vi "PRIME Detector Wait for Command to Complete.vi"(5 "Observation":T2={"Priority"=0, "ID"="", "Observer"="", "Obj Name"="", "Obj Type"="", "RA and DEC String"={"RA"="HH:MM:SS.nnn", "DEC"="DEG:arcmin:arcsec.nn"}, "Filters"=[], "Integration Time"=0.0, "Observation Status"=enum."Error", "Offsets"={"RA"=0.0, "DEC"=0.0, "ROT"=0.0}, "Images"=0, "Dither Options"={"Dither"=enum."None", "Dither Radius"=0.0, "Dither Points"=0, "Dither Phase"=0.0, "B Offset"={"RA"=0.0, "DEC"=0.0}}, "Comment 1"="", "Comment 2"=""}, 7 "Detector Config":T8={"Detector"=0, "Offsets"=[[0, 0, 0, 0, 0, 0, 0, 0, 0, 0, 0, 0, 0, 0, 0, 0, 0, 0, 0, 0, 0, 0, 0, 0, 0, 0, 0, 0, 0, 0, 0, 0]], "Detector Computer"={"Machine"="192.168.121.11", "Password"="rSL!nux23456", "FITS File Path"="", "Port"=44444, "Header Path"="", "Name"=""}, "FITS hdr template0"=path "", "FITS hdr template1"=path "", "FITS Data File Path"=path "", "FITS Detector Settings"={"Exp Time Short"=0.0, "# of Frames"=0.0, "Exp Time Long"=0.0, "# of Groups"=0.0, "Object Name"="", "Object"="", "Obs Type"="", "Image Type"="", "Observer"="", "Observer Affiliation"=""}, "Sim Folder"=path "", "Integration Mode"=enum."Ramp", "Integration Time"=0.0, "Frame Int Time"=0.0} {"Offsets" format="%04x"; "Detector" items=["0", "1", "2"]}, 8 "error in (no error)":errorcluster, 9 "Exp Time":dbl=60.0, 10 "timeout (120s)":dbl=120.0, 11 "connection ID":refnum<k5>) -> (0 "error out":errorcluster, 1 "Image Map":map{string, T1}(c390), 2 "Status":T13, 3 "connection ID out":refnum<k5>)   [LabVIEW 2024, in "PRIME Detector.lvclass"]
uses:
  PRIME Detector.lvclass
  PRIME Detector cluster Status.ctl
  RIMAS Detector Config.ctl
  RIMAS Detector Server Config.ctl
  RIMAS Observation Config.ctl
  Detector enum Detector Integration Mode.ctl
  typedefs/CC cluster Observation.ctl
  Observation Queue/CC enum Observation Status.ctl
  Telescope/CC cluster Telescope Offsets.ctl
  typedefs/CC cluster Observation Dither Options.ctl
  typedefs/CC enum Dither Selection.ctl
  typedefs/CC cluster RA and DEC.ctl
  Detector Image typedef cluster.ctl
  Detector Class.lvclass
panel:
  in  "Image List":T12
  out "Time Remaining":dbl(knob) scale=-1.0..30.0
  out "Command":string
  # "sec"
  # "sec"
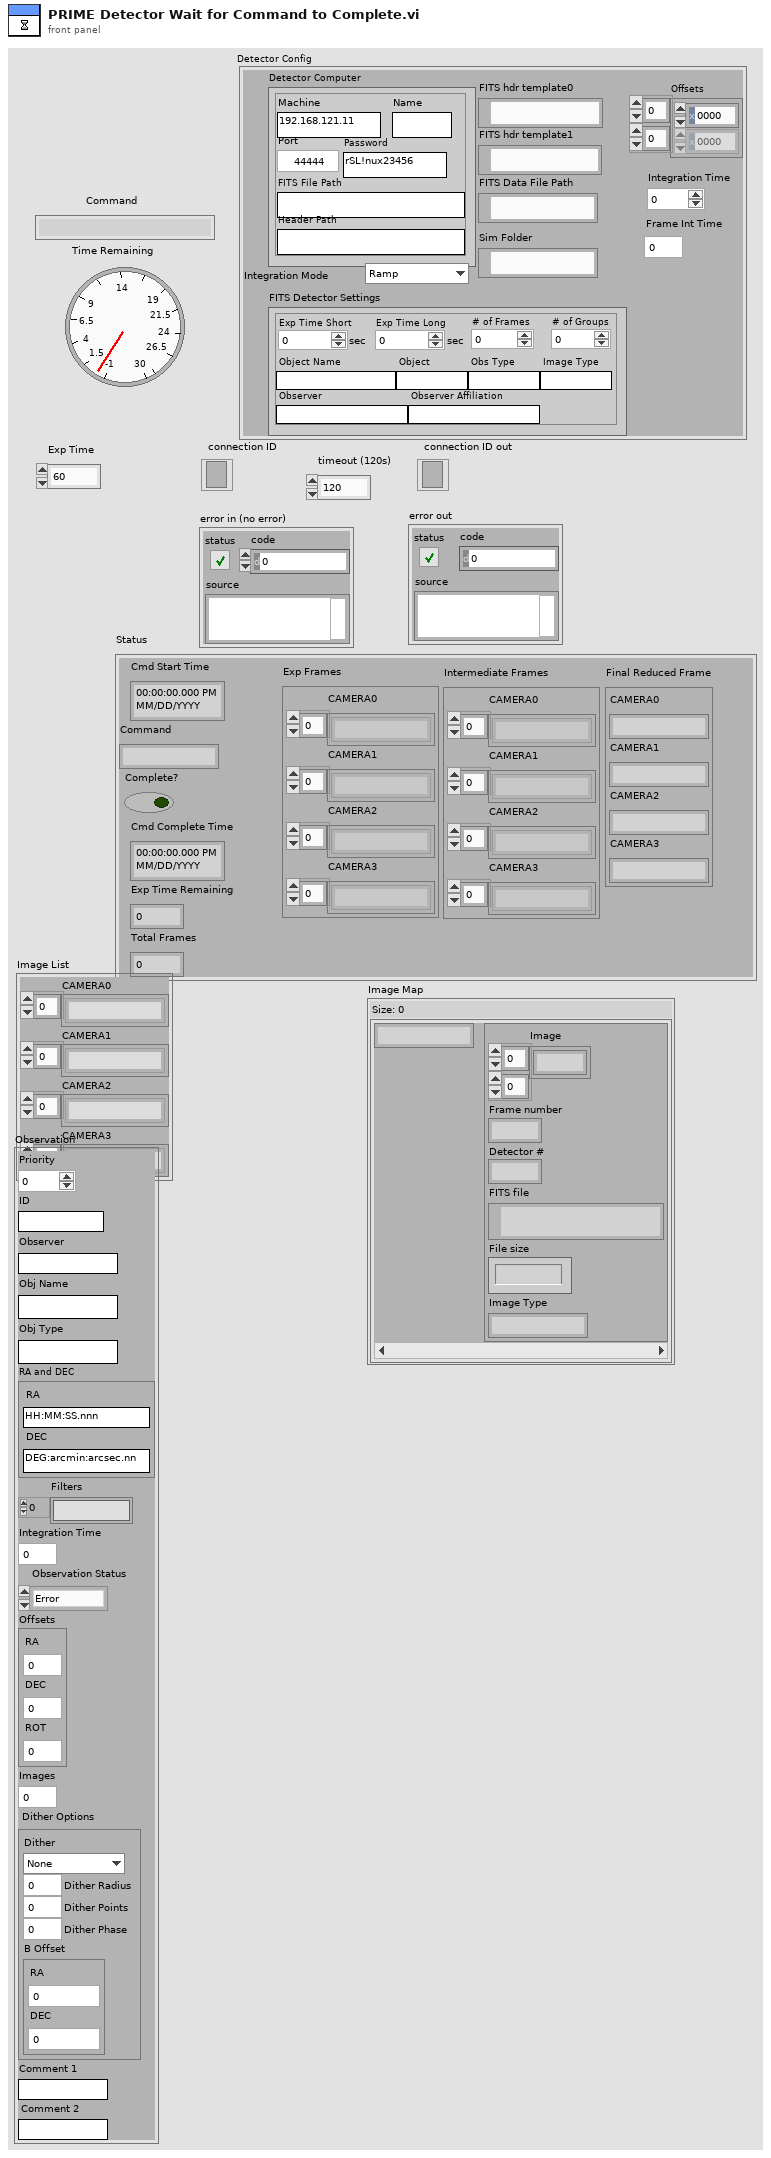
[diagram p1: front panel]
types:
  T1 = typedef "Detector Class.lvclass/Detector Image typedef cluster.ctl" = cluster{"Image":sgl[][], "Frame number":i32, "Detector #":u16, "FITS file":path, "File size":i64, "Image Type":string}
  T2 = typedef "CC cluster Observation.ctl" = cluster{"Priority":i32, "ID":string, "Observer":string, "Obj Name":string, "Obj Type":string, "RA and DEC String":cluster{"RA":string, "DEC":string}, "Filters":string[], "Integration Time":dbl, "Observation Status":T3, "Offsets":T4, "Images":i32, "Dither Options":T5, "Comment 1":string, "Comment 2":string}
  T3 = typedef "CC enum Observation Status.ctl" = enum16{"Ready", "Running", "Done", "Error"}
  T4 = typedef "CC cluster Telescope Offsets.ctl" = cluster{"RA":dbl, "DEC":dbl, "ROT":dbl}
  T5 = typedef "CC cluster Observation Dither Options.ctl" = cluster{"Dither":T6, "Dither Radius":dbl, "Dither Points":i32, "Dither Phase":dbl, "B Offset":T7}
  T6 = typedef "CC enum Dither Selection.ctl" = enum16{"None", "Circle", "Random", "ABBA"}
  T7 = typedef "CC cluster RA and DEC.ctl" = cluster{"RA":dbl, "DEC":dbl}
  T8 = typedef "RIMAS Detector Config.ctl" = cluster{"Detector":u16, "Offsets":u16[][], "Detector Computer":T9, "FITS hdr template0":path, "FITS hdr template1":path, "FITS Data File Path":path, "FITS Detector Settings":T10, "Sim Folder":path, "Integration Mode":T11, "Integration Time":dbl, "Frame Int Time":dbl}
  T9 = typedef "RIMAS Detector Server Config.ctl" = cluster{"Machine":string, "Password":string, "FITS File Path":string, "Port":u16, "Header Path":string, "Name":string}
  T10 = typedef "RIMAS Observation Config.ctl" = cluster{"Exp Time Short":dbl, "# of Frames":dbl, "Exp Time Long":dbl, "# of Groups":dbl, "Object Name":string, "Object":string, "Obs Type":string, "Image Type":string, "Observer":string, "Observer Affiliation":string}
  T11 = typedef "Detector enum Detector Integration Mode.ctl" = enum16{"Ramp", "CDS", "FOWLER2", "FOWLER4", "FOWLER8", "FOWLER16", "Raw"}
  T12 = cluster{"CAMERA0":string[], "CAMERA1":string[], "CAMERA2":string[], "CAMERA3":string[]}
  T13 = typedef "PRIME Detector cluster Status.ctl" = cluster{"Cmd Start Time":timestamp, "Command":string, "Complete?":bool, "Cmd Complete Time":timestamp, "Exp Time Remaining":dbl, "Total Frames":i32, "Exp Frames":cluster{"CAMERA0":string[], "CAMERA1":string[], "CAMERA2":string[], "CAMERA3":string[]}, "Intermediate Frames":cluster{"CAMERA0":string[], "CAMERA1":string[], "CAMERA2":string[], "CAMERA3":string[]}, "Final Reduced Frame":cluster{"CAMERA0":string, "CAMERA1":string, "CAMERA2":string, "CAMERA3":string}}
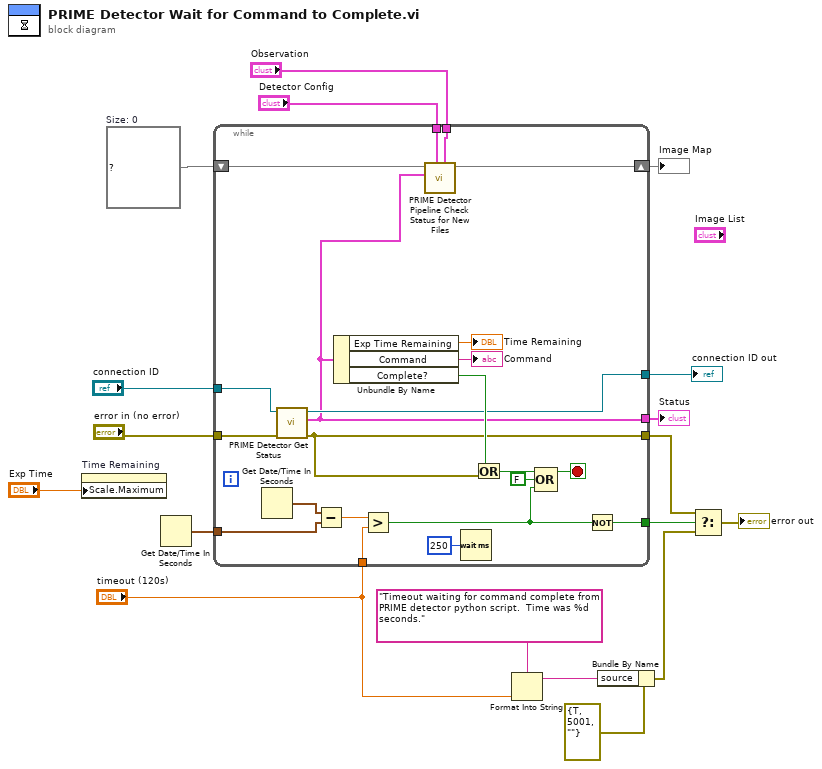
[diagram p0: block diagram]
diagram:
  w4 = map{string, T1} {}  # Size: 0
  n1 = property on="Time Remaining" class="Knob (strict)"("Scale.Maximum"="Exp Time") -> ()  [unwired: 2 in, 2 out]
  n2 = Get Date/Time In Seconds() -> (seconds since 1Jan1904=w16:timestamp)
  n3 = while {
    tunnel: "error in (no error)" -> [w40]
    tunnel: "connection ID" -> [w39]
    tunnel: [w36] -> w11
    tunnel: w16 -> [w33]
    tunnel: "timeout (120s)" -> [w31]
    tunnel: [w28] -> w14
    tunnel: [w22] -> w13
    tunnel: [w25] -> w12
    shift-right: [w23] -> w1
    shift-left: w4 -> [w24]
    tunnel: "Detector Config" -> [w21]
    tunnel: "Observation" -> [w20]
    stop <- w27 stop-if-true
    n4 = Get Date/Time In Seconds() -> (seconds since 1Jan1904=w34:timestamp)
    n5 = call "PRIME Detector Get Status.vi"("error in (no error)"=w40, "connection ID"=w39) -> ("error out"=w36:errorcluster, "Status"=w22:T13, "connection ID out"=w28:refnum<k5>)  [unwired: 6 in, 1 out]
    n6 = Subtract(x=w34, y=w33) -> (x-y=w32:dbl)
    n7 = Unbundle By Name(w22) -> ("Exp Time Remaining"=→"Time Remaining":dbl, "Command"=→"Command":string, "Complete?"=w38:bool)
    n8 = Greater?(x=w32, y=w31) -> (0:w26:bool)
    n9 = call "PRIME Detector Pipeline Check Status for New Files.vi"("Observation"=w20, "Detector Config"=w21, "Status"=w22, "Map in"=w24) -> ("Map out"=w23:map{string, T1})  [unwired: 6 in, 1 out]
    n10 = Wait (ms)(milliseconds to wait=u32 250 ("millisecond multiple")) -> ()  [unwired: 1 out]
    n11 = Or(x=w38, y=w36) -> (x .or. y?=w37:bool)
    n12 = Compound Arithmetic op=OR(w37, FALSE ("value"), w26) -> (w27:bool)
    n13 = Not(x=w26) -> (.not. x?=w25:bool)
  }
  "connection ID out" <- w14
  "Status" <- w13
  "Image Map" <- w1
  n14 = Format Into String(format string="Timeout waiting for command complete from PRIME detector python script.  Time was %d seconds." ("source"), "timeout (120s)") -> (resulting string=w6:string)  [unwired: 2 in, 1 out]
  n15 = Bundle By Name(cluster=errorcluster {"status"=TRUE, "code"=5001, "source"=""} ("f"), "source"=w6) -> (w5:errorcluster)
  n16 = Select(t=w11, s=w12, f=w5) -> (s? t:f=→"error out":errorcluster)
